vi "thermistor_reduced_param_init.vi"() -> ()   [LabVIEW 2018]
panel:
  out "Init Data Out":fxp<+,32,16>[](array[numeric])
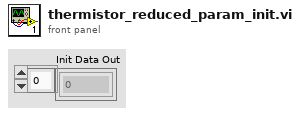
[diagram p1: front panel]
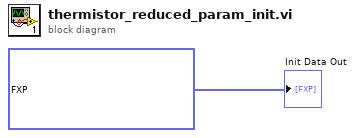
[diagram p0: block diagram]
diagram:
  "Init Data Out" <- fxp<+,32,16>[] [3434.0, 0.099517822265625, 3977.0, 0.01611328125]
